vi "TDK释放.vi"(9 "error out":errorcluster, 10 "VISA resource name out":refnum<visa-resource-name>, 11 "Globalize (0: Single)":u16) -> (2 "error out 2":errorcluster caption="error out", 3 "VISA resource name out 2":refnum<visa-resource-name>)   [LabVIEW 2021]
uses:
  <instrlib>/TDK-Lambda G Series/TDK-Lambda G Series.lvlib
panel:
  in  "停止":bool
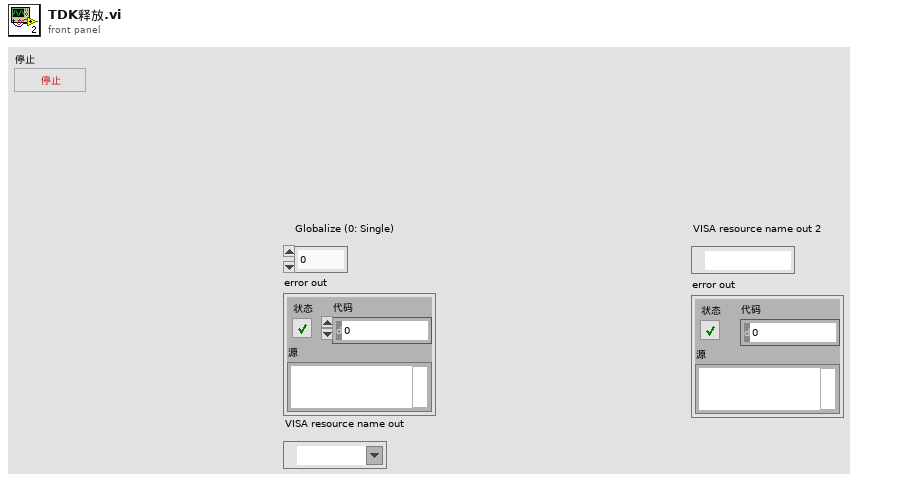
[diagram p1: front panel]
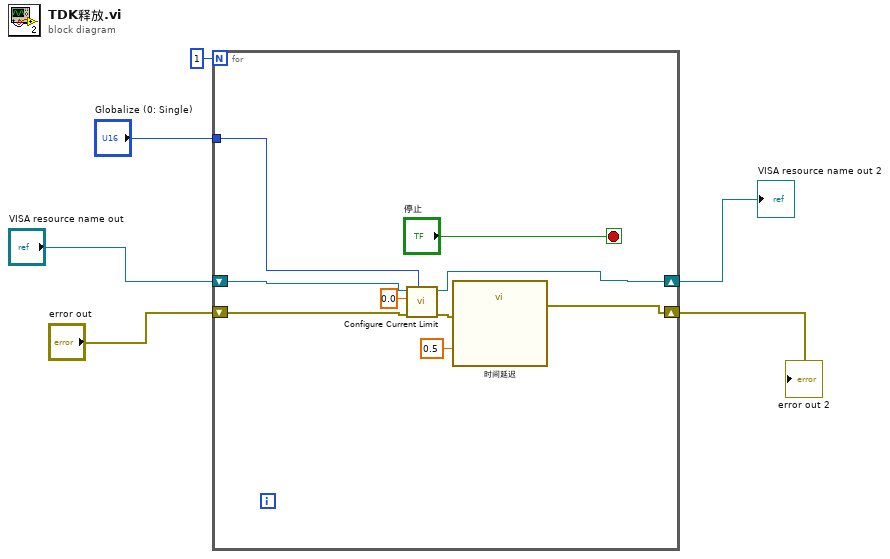
[diagram p0: block diagram]
diagram:
  n1 = for {
    N: 1 -> [_]
    shift-right: [w11] -> w3
    shift-left: "VISA resource name out" -> [w15]
    shift-right: [w10] -> w2
    shift-left: "error out" -> [w14]
    tunnel: "Globalize (0: Single)" -> [w13]
    stop <- "停止" stop-if-true
    n2 = call <instrlib>:"Configure Current Limit.vi"("Globalize (0: Single)"=w13, "error in (no error)"=w14, "Current Limit (0A)"=0.0, "VISA resource name"=w15) -> ("error out"=w9:errorcluster, "VISA resource name out"=w11:refnum<visa-resource-name>)  [unwired: 6 in]
    n3 = call "时间延迟"("error in (no error)"=w9, "Delay Time (s)"=0.5) -> ("error out"=w10:errorcluster)  [unwired: 9 in]
  }
  "VISA resource name out 2" <- w3
  "error out 2" <- w2
